vi "Lissajous_curves.vi"() -> ()   [LabVIEW 2022 SP3]
uses:
  <vilib>/measure/NI_MABase.lvlib
panel:
  in  "stop":bool
  in  "Equal Freq":bool
  in  "Tab Control":enum32{"WaveF Graph", "XY Graph"}(tab)
  out "Waveform Graph":dynamicdata(graph)
  out "XY Graph":cluster{"Y":dbl[], "Y":dbl[]}(graph)
  in  "Frequency":dbl(knob)=10.0 scale=0.0..50.0
  in  "Phase":dbl(knob) scale=0.0..180.0
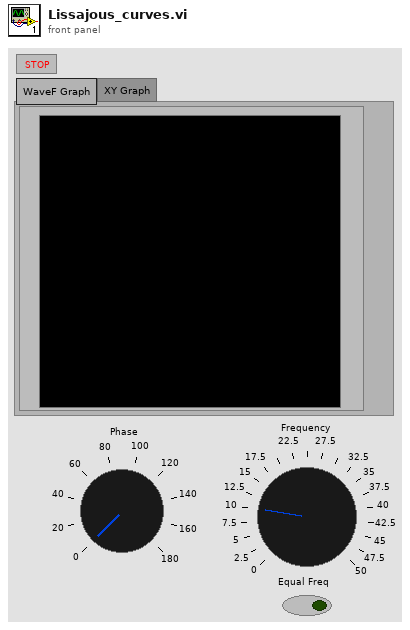
[diagram p1: front panel]
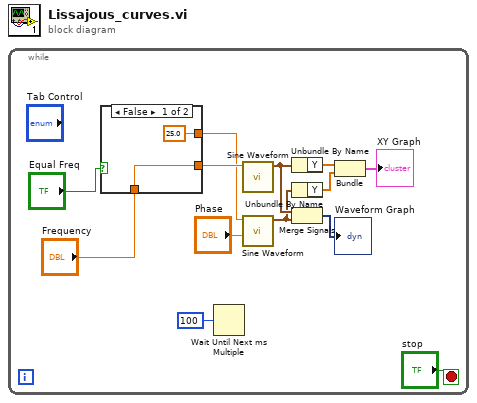
[diagram p0: block diagram]
diagram:
  n1 = while {
    stop <- "stop" stop-if-true
    n2 = case shown="False" "Equal Freq" {
      tunnel: [w15 w16] -> w5
      tunnel: "Frequency" -> [w15 w16]
      tunnel: [25.0 ("Frequency") w16] -> w3
      frame False {
      }
      frame True {
      }
    }
    n3 = Wait Until Next ms Multiple(millisecond multiple=u32 100) -> ()  [unwired: 1 out]
    n4 = call <vilib>:"Sine Waveform.vi"("frequency"=w5) -> ("signal out"=w9:waveform(dbl))  [unwired: 9 in, 1 out]
    n5 = call <vilib>:"Sine Waveform.vi"("phase"="Phase", "frequency"=w3) -> ("signal out"=w8:waveform(dbl))  [unwired: 8 in, 1 out]
    n6 = Unbundle By Name(w9) -> ("Y"=w11:dbl[])
    n7 = Unbundle By Name(w8) -> ("Y"=w10:dbl[])
    n8 = Merge Signals(w9, w8) -> (→"Waveform Graph":dynamicdata)
    n9 = Bundle("Y"=w11, "Y"=w10) -> (→"XY Graph":cluster{"Y":dbl[], "Y":dbl[]})  [unwired: 1 in]
  }
